vi "assi_state_driver.vi"(1 "ASSI Signal":dbl) -> (0 "ASSI State":string)   [LabVIEW 2017]
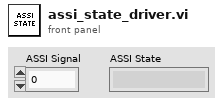
[diagram p1: front panel]
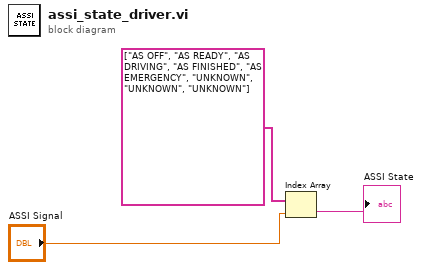
[diagram p0: block diagram]
diagram:
  n1 = Index Array(array=string[] ["AS OFF", "AS READY", "AS DRIVING", "AS FINISHED", "AS EMERGENCY", "UNKNOWN", "UNKNOWN", "UNKNOWN"], index="ASSI Signal") -> (element=→"ASSI State":string)
